vi "Connect and setup SMU.vi"(8 "error in (no error)":errorcluster, 11 "VISA refnum in":refnum<visa-resource-name>) -> (0 "error out":errorcluster, 2 "Resistance":dbl, 3 "VISA refnum out":refnum<visa-resource-name>)   [LabVIEW 2021]
uses:
  <instrlib>/Keithley 2450/Keithley 2450.lvlib
  controls/SMU settings.ctl
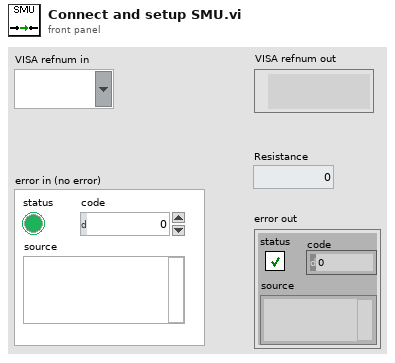
[diagram p1: front panel]
types:
  T1 = typedef "SMU settings.ctl" = cluster{"Source Mode ":u16, "Source Level":dbl, "Source Limit":dbl, "Measure Function":u16, "Remote sense":bool, "Clear buffer?":bool, "Beep":bool, "High Capacity":bool, "Terminals":u16, "PLCs":dbl, "Fast measurement":bool}
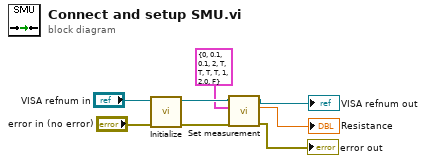
[diagram p0: block diagram]
diagram:
  n1 = call <instrlib>:"Initialize.vi"("error in (no error)"="error in (no error)", "VISA resource name"="VISA refnum in") -> ("error out"=w5:errorcluster, "VISA resource name out"=w6:refnum<visa-resource-name>)  [unwired: 8 in]
  n2 = call "Set measurement.vi"("error in (no error)"=w5, "Measurement settings"=T1 {"Source Mode "=0, "Source Level"=0.1, "Source Limit"=0.1, "Measure Function"=2, "Remote sense"=TRUE, "Clear buffer?"=TRUE, "Beep"=TRUE, "High Capacity"=TRUE, "Terminals"=1, "PLCs"=2.0, "Fast measurement"=FALSE}, "VISA resource name"=w6) -> ("error out"=→"error out":errorcluster, "Value"=→"Resistance":dbl, "VISA resource name out"=→"VISA refnum out":refnum<visa-resource-name>)  [unwired: 4 in, 2 out]
